vi "5492_CollectMotor.vi"(0 "MotorControlDevRef":T1={"DeviceStatus"={"status"=FALSE, "code"=0, "source"=""}, "Type"=enum."PWM", "PWM"={"PWM Channel"=enum."Invalid", "DeadBand"={"Name"="", "maxPositivePwm"=0, "minPositivePwm"=0, "centerPwm"=0, "maxNegativePwm"=0, "minNegativePwm"=0, "angularRange"=0}}, "CAN"={"Device Number"=0, "SetOutput VI Ref"=variant(enum8{"Percent VBus", "Current", "Speed", "Position", "Voltage"} enum."Percent VBus"), "GetOutput VI Ref"=variant(refnum<k1> refnum), "Enable VI Ref"=variant(dbl 12.0), "Disable VI Ref"=variant(enum8{"Percent VBus", "Speed", "Position", "Slave", "Unchanged / Invalid", "Voltage Compensation", "Current", "Motion Profile"} enum."Percent VBus"), "Data"=variant}, "Invert"=FALSE, "DIO PWM"={"PWM \"Enable\" Channel"=enum."Invalid", "DIOChannel"=enum."Invalid", "PWM Rate"=0.0}}, 1 "Wait Start In":dbl, 5 "Limit Switch PhoenixMotorControlDevRef":T1={"DeviceStatus"={"status"=FALSE, "code"=0, "source"=""}, "Type"=enum."PWM", "PWM"={"PWM Channel"=enum."Invalid", "DeadBand"={"Name"="", "maxPositivePwm"=0, "minPositivePwm"=0, "centerPwm"=0, "maxNegativePwm"=0, "minNegativePwm"=0, "angularRange"=0}}, "CAN"={"Device Number"=0, "SetOutput VI Ref"=variant(enum8{"Percent VBus", "Current", "Speed", "Position", "Voltage"} enum."Percent VBus"), "GetOutput VI Ref"=variant(refnum<k1> refnum), "Enable VI Ref"=variant(dbl 12.0), "Disable VI Ref"=variant(enum8{"Percent VBus", "Speed", "Position", "Slave", "Unchanged / Invalid", "Voltage Compensation", "Current", "Motion Profile"} enum."Percent VBus"), "Data"=variant}, "Invert"=FALSE, "DIO PWM"={"PWM \"Enable\" Channel"=enum."Invalid", "DIOChannel"=enum."Invalid", "PWM Rate"=0.0}}, 7 "Spit":bool, 9 "Collect":bool, 11 "Setting":string, 12 "Loop Iteration":dbl) -> (4 "MotorControlDevRef 2":T1={"DeviceStatus"={"status"=FALSE, "code"=0, "source"=""}, "Type"=enum."PWM", "PWM"={"PWM Channel"=enum."Invalid", "DeadBand"={"Name"="", "maxPositivePwm"=0, "minPositivePwm"=0, "centerPwm"=0, "maxNegativePwm"=0, "minNegativePwm"=0, "angularRange"=0}}, "CAN"={"Device Number"=0, "SetOutput VI Ref"=variant(enum8{"Percent VBus", "Current", "Speed", "Position", "Voltage"} enum."Percent VBus"), "GetOutput VI Ref"=variant(refnum<k1> refnum), "Enable VI Ref"=variant(dbl 12.0), "Disable VI Ref"=variant(enum8{"Percent VBus", "Speed", "Position", "Slave", "Unchanged / Invalid", "Voltage Compensation", "Current", "Motion Profile"} enum."Percent VBus"), "Data"=variant}, "Invert"=FALSE, "DIO PWM"={"PWM \"Enable\" Channel"=enum."Invalid", "DIOChannel"=enum."Invalid", "PWM Rate"=0.0}}, 6 "Wait Start Out":dbl, 15 "Setting but Out":string)   [LabVIEW 2017]
uses:
  <vilib>/Rock Robotics/WPI/MotorControl/WPI_MotorControlDeviceRef.ctl
  <vilib>/Rock Robotics/WPI/MotorControl/WPI_MotorControlType.ctl
  <vilib>/Rock Robotics/SystemInterfaces/DIO/FPGA_DIOPWMChannel.ctl
  <vilib>/Rock Robotics/WPI/PWM/WPI_PWMDeadband.ctl
  <vilib>/Rock Robotics/SystemInterfaces/DIO/FPGA_DIOChannel.ctl
  Public/Documents/Cross The Road Electronics/Phoenix-LabVIEW/Motor Controller/Controls/CTRE_Phoenix_MotorControl_ControlMode.ctl
  <vilib>/Rock Robotics/WPI/MotorControl/WPI_MotorControlSafetyCheck.vi
  Public/Documents/Cross The Road Electronics/Phoenix-LabVIEW/Motor Controller/Get/CTRE_Phoenix_MotorController_GetAnalogData.vi
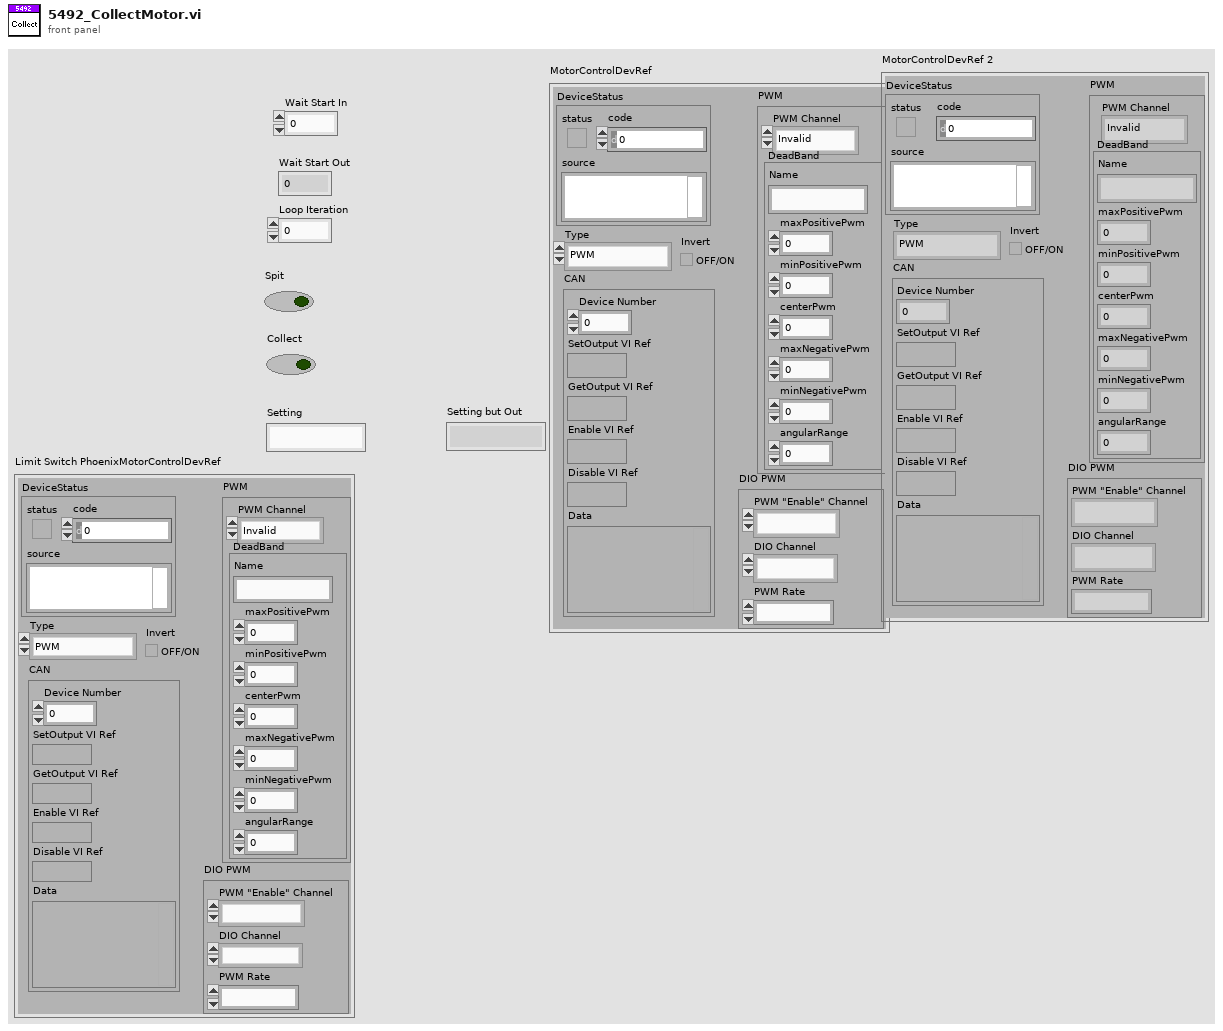
[diagram p1: front panel]
types:
  T1 = typedef "WPI_MotorControlDeviceRef.ctl" = cluster{"DeviceStatus":errorcluster, "Type":T2, "PWM":cluster{"PWM Channel":T3, "DeadBand":T4}, "CAN":cluster{"Device Number":u8, "SetOutput VI Ref":variant, "GetOutput VI Ref":variant, "Enable VI Ref":variant, "Disable VI Ref":variant, "Data":variant}, "Invert":bool, "DIO PWM":cluster{"PWM \"Enable\" Channel":T3, "DIOChannel":T5, "PWM Rate":dbl}}
  T2 = typedef "WPI_MotorControlType.ctl" = enum16{"PWM", "CAN", "DIO PWM"}
  T3 = typedef "FPGA_DIOPWMChannel.ctl" = enum8{"PWM 0", "PWM 1", "PWM 2", "PWM 3", "PWM 4", "PWM 5", "PWM 6", "PWM 7", "PWM 8", "PWM 9", "PWM MXP 0", "PWM MXP 1", "PWM MXP 2", "PWM MXP 3", "PWM MXP 4", "PWM MXP 5", "PWM MXP 6", "PWM MXP 7", "PWM MXP 8", "PWM MXP 9", "Invalid"}
  T4 = typedef "WPI_PWMDeadband.ctl" = cluster{"Name":string, "maxPositivePwm":i32, "minPositivePwm":i32, "centerPwm":i32, "maxNegativePwm":i32, "minNegativePwm":i32, "angularRange":u16}
  T5 = typedef "FPGA_DIOChannel.ctl" = enum8{"DIO 0", "DIO 1", "DIO 2", "DIO 3", "DIO 4", "DIO 5", "DIO 6", "DIO 7", "DIO 8", "DIO 9", "DIO MXP 0", "DIO MXP 1", "DIO MXP 2", "DIO MXP 3", "DIO MXP 4", "DIO MXP 5", "DIO MXP 6", "DIO MXP 7", "DIO MXP 8", "DIO MXP 9", "DIO MXP 10", "DIO MXP 11", "DIO MXP 12", "DIO MXP 13", "DIO MXP 14", "DIO MXP 15", "SPI Port CS1", "SPI Port CS2", "SPI Port CS3", "SPI Port MISO", "SPI Port MOSI", "Invalid"}
  T6 = typedef "CTRE_Phoenix_MotorControl_ControlMode.ctl" = u16
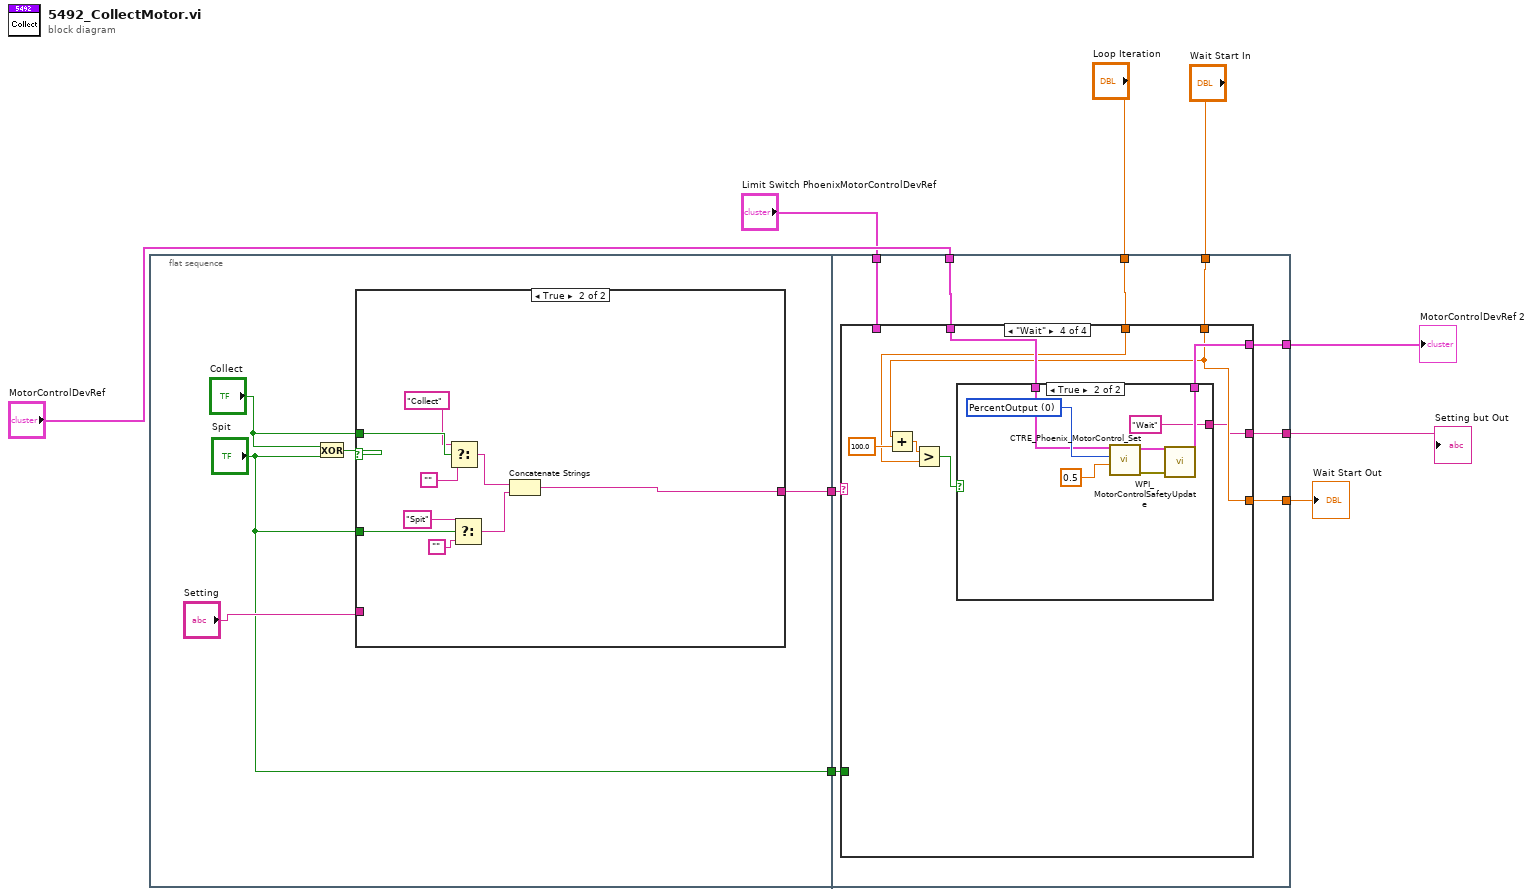
[diagram p0: block diagram]
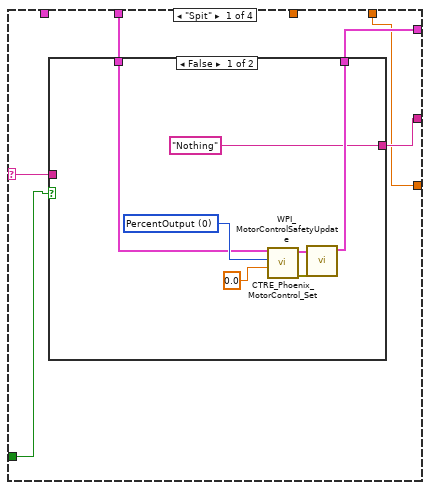
[diagram p3: hidden frame]
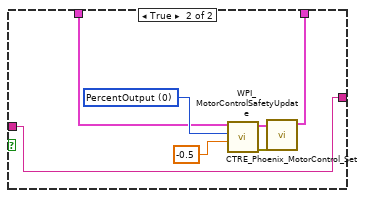
[diagram p4: hidden frame]
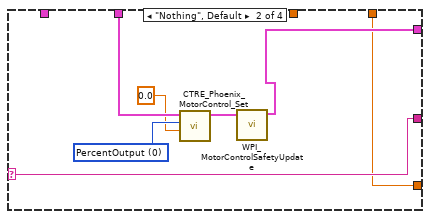
[diagram p5: hidden frame]
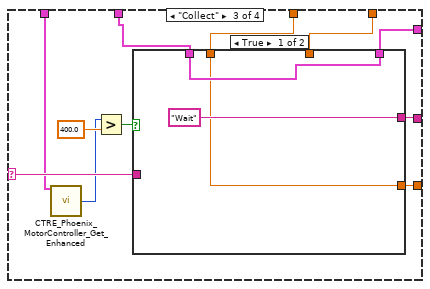
[diagram p6: hidden frame]
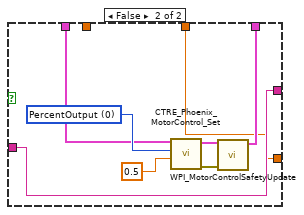
[diagram p7: hidden frame]
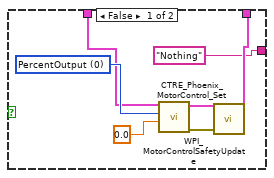
[diagram p8: hidden frame]
diagram:
  n1 = flat-sequence {
    tunnel: [w11] -> w9
    tunnel: ["Spit"] -> w5
    tunnel: w9 -> [w33]
    tunnel: [w25] -> w8
    tunnel: "MotorControlDevRef" -> [w32]
    tunnel: [w31] -> w6
    tunnel: w5 -> [w30]
    tunnel: "Limit Switch PhoenixMotorControlDevRef" -> [w29]
    tunnel: "Loop Iteration" -> [w28]
    tunnel: [w27] -> w2
    tunnel: "Wait Start In" -> [w26]
    frame #0 {
      n2 = Exclusive Or(1:"Spit", 2:"Collect") -> (0:w14:bool)
      n3 = case shown="True" w14 {
        tunnel: "Collect" -> [_ w22]
        tunnel: "Spit" -> [_ w20]
        tunnel: "Setting" -> [w15 _]
        tunnel: [w15 w16] -> w11
        frame False {
        }
        frame True {
          n4 = Select(t="Collect", s=w22, f="") -> (s? t:f=w23:string)
          n5 = Select(t="Spit", s=w20, f="") -> (s? t:f=w17:string)
          n6 = Concatenate Strings(w23, w17) -> (w16:string)
        }
      }
    }
    frame #1 {
      n7 = case shown="\"Wait\"" w33 {
        selector: w33 -> [w35 w60 w69 _]
        tunnel: [w36 w60 w70 w83] -> w25
        tunnel: w32 -> [w38 w58 w68 w90]
        tunnel: [w39 w59 w71 w89] -> w31
        tunnel: w30 -> [w37 _ _ _]
        tunnel: w29 -> [_ _ w67 _]
        tunnel: w28 -> [_ _ w66 w84]
        tunnel: [w34 w54 w65 w86] -> w27
        tunnel: w26 -> [w34 w54 w64 w86]
        frame "Spit" {
          n8 = case shown="False" w37 {
            tunnel: [w41 w49] -> w39
            tunnel: w38 -> [w42 w48]
            tunnel: ["Nothing" w47] -> w36
            tunnel: w35 -> [_ w47]
            frame False {
              w45 = T6 0 items=["PercentOutput"=0, "Position"=1, "Velocity"=2, "Current"=3, "Follower"=5, "MotionProfile"=6, "MotionMagic"=7, "MotionMagicArc"=8, "MotionProfileArc"=10, "Disabled"=15] ("Control Mode")
              n9 = call "CTRE_Phoenix_MotorControl_Set.vi"("Output"=0.0, "Control Mode"=w45, "PhoenixMotorControlDevRef"=w42) -> ("error out"=w44:errorcluster, "PhoenixMotorControlDevRef"=w43:T1)  [unwired: 7 in]
              n10 = call <vilib>:"WPI_MotorControlSafetyUpdate.vi"("error in (no error)"=w44, "MotorControlDevRef"=w43) -> ("MotorControlDevRef"=w41:T1)  [unwired: 9 out]
            }
            frame True {
              w52 = T6 0 items=["PercentOutput"=0, "Position"=1, "Velocity"=2, "Current"=3, "Follower"=5, "MotionProfile"=6, "MotionMagic"=7, "MotionMagicArc"=8, "MotionProfileArc"=10, "Disabled"=15] ("Control Mode")
              n11 = call "CTRE_Phoenix_MotorControl_Set.vi"("Output"=-0.5, "Control Mode"=w52, "PhoenixMotorControlDevRef"=w48) -> ("error out"=w51:errorcluster, "PhoenixMotorControlDevRef"=w50:T1)  [unwired: 7 in]
              n12 = call <vilib>:"WPI_MotorControlSafetyUpdate.vi"("error in (no error)"=w51, "MotorControlDevRef"=w50) -> ("MotorControlDevRef"=w49:T1)  [unwired: 9 out]
            }
          }
        }
        frame "Nothing", Default {
          w56 = T6 0 items=["PercentOutput"=0, "Position"=1, "Velocity"=2, "Current"=3, "Follower"=5, "MotionProfile"=6, "MotionMagic"=7, "MotionMagicArc"=8, "MotionProfileArc"=10, "Disabled"=15] ("Control Mode")
          n13 = call "CTRE_Phoenix_MotorControl_Set.vi"("Output"=0.0, "Control Mode"=w56, "PhoenixMotorControlDevRef"=w58) -> ("PhoenixMotorControlDevRef"=w57:T1)  [unwired: 7 in, 1 out]
          n14 = call <vilib>:"WPI_MotorControlSafetyUpdate.vi"("MotorControlDevRef"=w57) -> ("MotorControlDevRef"=w59:T1)  [unwired: 1 in, 9 out]
        }
        frame "Collect" {
          n15 = call-poly "CTRE_Phoenix_MotorController_Get_Enhanced.vi"("PhoenixMotorControlDevRef"=w67) -> ("AnalogInRaw"=w61:i32)  [unwired: 10 in, 4 out]
          n16 = Greater?(x=w61, y=400.0) -> (0:w63:bool)
          n17 = case shown="True" w63 {
            tunnel: [w73 w78] -> w71
            tunnel: w68 -> [w73 w77]
            tunnel: ["Wait" w76] -> w70
            tunnel: w69 -> [_ w76]
            tunnel: w66 -> [w72 _]
            tunnel: [w72 w75] -> w65
            tunnel: w64 -> [_ w75]
            frame True {
            }
            frame False {
              w82 = T6 0 items=["PercentOutput"=0, "Position"=1, "Velocity"=2, "Current"=3, "Follower"=5, "MotionProfile"=6, "MotionMagic"=7, "MotionMagicArc"=8, "MotionProfileArc"=10, "Disabled"=15] ("Control Mode")
              n18 = call "CTRE_Phoenix_MotorControl_Set.vi"("Output"=0.5, "Control Mode"=w82, "PhoenixMotorControlDevRef"=w77) -> ("error out"=w80:errorcluster, "PhoenixMotorControlDevRef"=w79:T1)  [unwired: 7 in]
              n19 = call <vilib>:"WPI_MotorControlSafetyUpdate.vi"("error in (no error)"=w80, "MotorControlDevRef"=w79) -> ("MotorControlDevRef"=w78:T1)  [unwired: 9 out]
            }
          }
        }
        frame "Wait" {
          n20 = Add(x=w86, y=100.0) -> (x+y=w87:dbl)
          n21 = Greater?(x=w87, y=w84) -> (0:w88:bool)
          n22 = case shown="True" w88 {
            tunnel: w90 -> [w93 w100]
            tunnel: [w92 w99] -> w89
            tunnel: ["Nothing" "Wait"] -> w83
            frame False {
              w97 = T6 0 items=["PercentOutput"=0, "Position"=1, "Velocity"=2, "Current"=3, "Follower"=5, "MotionProfile"=6, "MotionMagic"=7, "MotionMagicArc"=8, "MotionProfileArc"=10, "Disabled"=15] ("Control Mode")
              n23 = call "CTRE_Phoenix_MotorControl_Set.vi"("Output"=0.0, "Control Mode"=w97, "PhoenixMotorControlDevRef"=w93) -> ("error out"=w95:errorcluster, "PhoenixMotorControlDevRef"=w94:T1)  [unwired: 7 in]
              n24 = call <vilib>:"WPI_MotorControlSafetyUpdate.vi"("error in (no error)"=w95, "MotorControlDevRef"=w94) -> ("MotorControlDevRef"=w92:T1)  [unwired: 9 out]
            }
            frame True {
              w104 = T6 0 items=["PercentOutput"=0, "Position"=1, "Velocity"=2, "Current"=3, "Follower"=5, "MotionProfile"=6, "MotionMagic"=7, "MotionMagicArc"=8, "MotionProfileArc"=10, "Disabled"=15] ("Control Mode")
              n25 = call "CTRE_Phoenix_MotorControl_Set.vi"("Output"=0.5, "Control Mode"=w104, "PhoenixMotorControlDevRef"=w100) -> ("error out"=w102:errorcluster, "PhoenixMotorControlDevRef"=w101:T1)  [unwired: 7 in]
              n26 = call <vilib>:"WPI_MotorControlSafetyUpdate.vi"("error in (no error)"=w102, "MotorControlDevRef"=w101) -> ("MotorControlDevRef"=w99:T1)  [unwired: 9 out]
            }
          }
        }
      }
    }
  }
  "Setting but Out" <- w8
  "MotorControlDevRef 2" <- w6
  "Wait Start Out" <- w2
